vi "Write_LED.vi"(0 "COM Bluegiga in":refnum<visa-resource-name>, 1 "Handle table":string[][](array[string]), 2 "Registro Completo":u8[](array[numeric]), 4 "Modo":u8, 6 "Color (constant)":u32(colorbox), 7 "error in (no error)":errorcluster, 8 "Intensidad (One Shot)":u8, 9 "Color (Breathe)":u8, 10 "Color (One Shot)":u8, 11 "Intensidad (breathe)":u8, 13 "Delay (breathe)":u16, 14 "Service UUID":string, 16 "Characteristic UUID":string, 17 "Connection Status":T1={"MAC Address"="", "cnx handle"=0, "cnx flags"=0, "Address Type"=125, "Connection Interval (ms)"=125, "Timeout(ms)"=125, "Latency"=0, "bonding handle"=0} {"Address Type" items=["Public", "Random"]}) -> (20 "COM Bluegiga out":refnum<visa-resource-name>, 27 "error out":errorcluster)   [LabVIEW 2020]
uses:
  <vilib>/BLE/type_def/connection_status_bundle.ctl
  <vilib>/BLE/type_def/address_type.ctl
  <vilib>/BLE/ble_functions/ble_write_by_service_characteristic_uint8array.vi
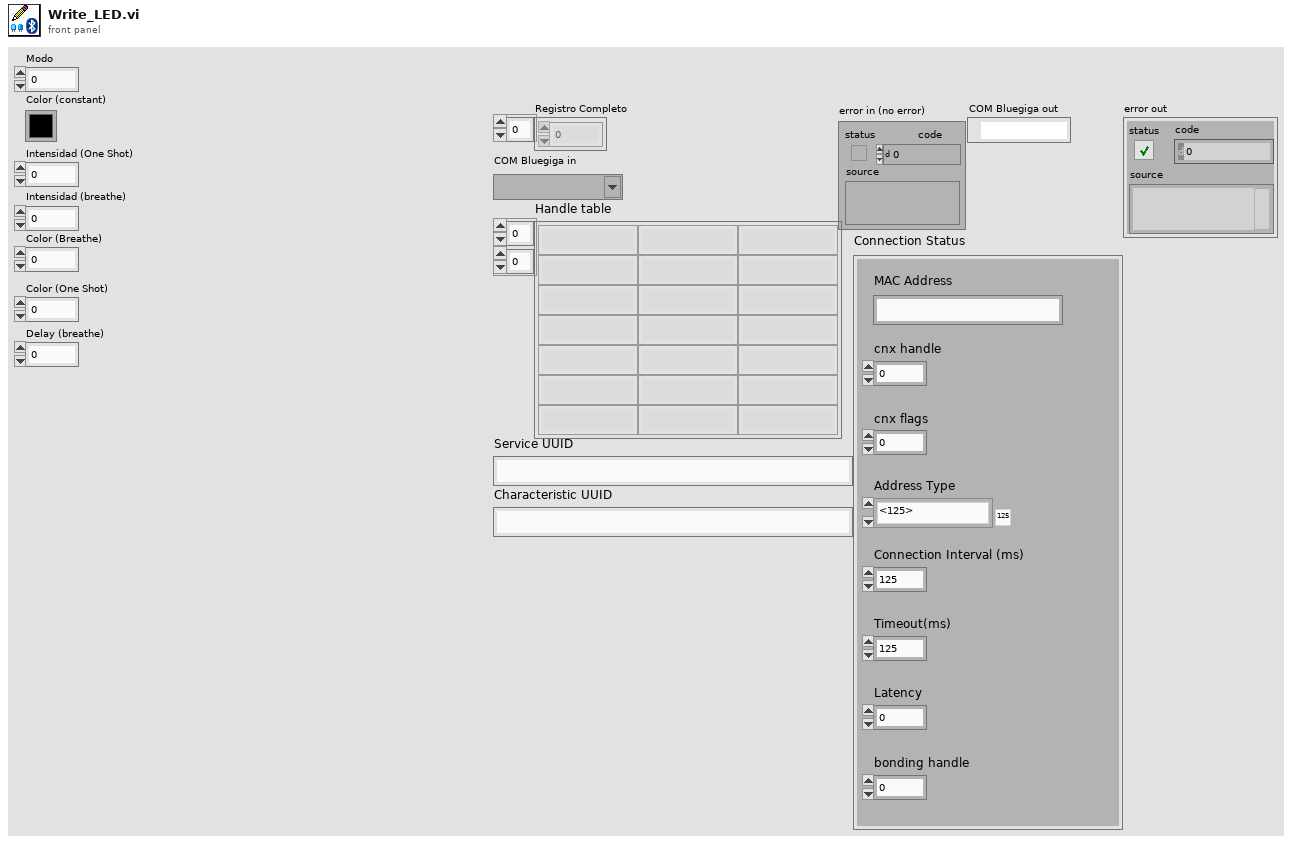
[diagram p1: front panel]
types:
  T1 = typedef "connection_status_bundle.ctl" = cluster{"MAC Address":string, "cnx handle":u8, "cnx flags":u8, "Address Type":T2, "Connection Interval (ms)":u16, "Timeout(ms)":u16, "Latency":u16, "bonding handle":u8}
  T2 = typedef "address_type.ctl" = u8
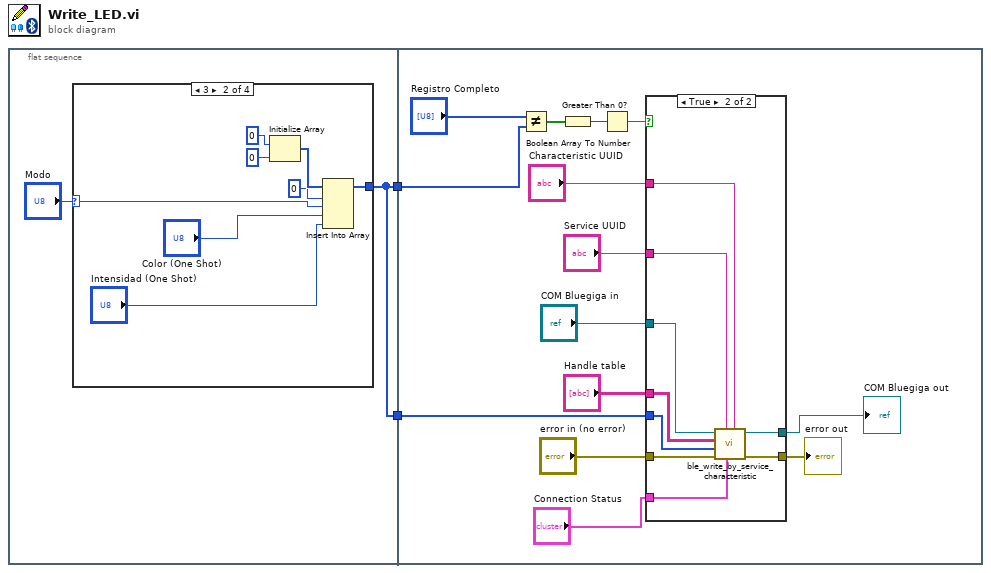
[diagram p0: block diagram]
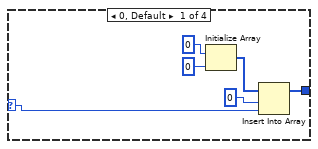
[diagram p2: hidden frame]
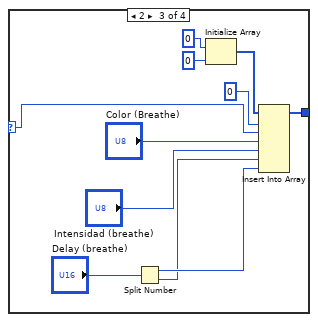
[diagram p3: hidden frame]
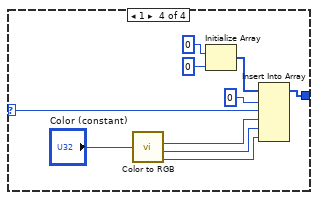
[diagram p4: hidden frame]
diagram:
  n1 = flat-sequence {
    tunnel: [w3] -> w2
    tunnel: [w3] -> w1
    tunnel: w2 -> [w41]
    tunnel: w1 -> [w40]
    frame #0 {
      n2 = case shown="3" "Modo" {
        selector: "Modo" -> [w6 w14 w25 w34]
        tunnel: [w5 w13 w19 w30] -> w3
        frame 0, Default {
          n3 = Initialize Array(u8 0 ("element"), 0 ("dimension size")) -> (w10:u8[])
          n4 = Insert Into Array(array=w10, index=0, new element=w6) -> (w5:u8[])
        }
        frame 3 {
          n5 = Initialize Array(u8 0 ("element"), 0 ("dimension size")) -> (w18:u8[])
          n6 = Insert Into Array(array=w18, index=0, new element #1=w14, new element #2="Color (One Shot)", new element #3="Intensidad (One Shot)") -> (w13:u8[])
        }
        frame 2 {
          n7 = Split Number(x="Delay (breathe)") -> (hi(x)=w21:u8, lo(x)=w20:u8)
          n8 = Initialize Array(u8 0 ("element"), 0 ("dimension size")) -> (w29:u8[])
          n9 = Insert Into Array(array=w29, index=0, new element #1=w25, new element #2="Color (Breathe)", new element #3="Intensidad (breathe)", new element #4=w20, new element #5=w21) -> (w19:u8[])
        }
        frame 1 {
          n10 = call <vilib>:"Color to RGB.vi"("Color"="Color (constant)") -> ("R"=w33:u8, "G"=w32:u8, "B"=w31:u8)  [unwired: 1 out]
          n11 = Initialize Array(u8 0 ("element"), 0 ("dimension size")) -> (w39:u8[])
          n12 = Insert Into Array(array=w39, index=0, new element #1=w34, new element #2=w33, new element #3=w32, new element #4=w31) -> (w30:u8[])
        }
      }
    }
    frame #1 {
      n13 = Not Equal?(x="Registro Completo", y=w40) -> (x != y?=w52:bool[])
      n14 = Boolean Array To Number(Boolean array=w52) -> (number=w53:u32)
      n15 = Greater Than 0?(x=w53) -> (x > 0?=w51:bool)
      n16 = case shown="True" w51 {
        tunnel: [w54 w64] -> w46
        tunnel: [w55 w63] -> w47
        tunnel: "COM Bluegiga in" -> [w55 w62]
        tunnel: "Handle table" -> [_ w61]
        tunnel: "error in (no error)" -> [w54 w60]
        tunnel: "Connection Status" -> [_ w59]
        tunnel: "Service UUID" -> [_ w58]
        tunnel: "Characteristic UUID" -> [_ w57]
        tunnel: w41 -> [_ w56]
        frame False {
        }
        frame True {
          n17 = call-poly <vilib>:"ble_write_by_service_characteristic.vi"("Characteristic UUID"=w57, "Connection Status"=w59, "Service UUID"=w58, "error in (no error)"=w60, "data"=w56, "Handle table"=w61, "COM Bluegiga in"=w62) -> ("error out"=w64:errorcluster, "COM Bluegiga out"=w63:refnum<visa-resource-name>)  [unwired: 3 in]
        }
      }
      "COM Bluegiga out" <- w47
      "error out" <- w46
    }
  }
